vi "TwoPointCaculateAngle.vi"(2 "Point 2":cluster{"X":dbl, "Y":dbl}, 3 "Point 1":cluster{"X":dbl, "Y":dbl}) -> (0 "©·«×":dbl, 1 "deg( «×)":dbl)   [LabVIEW 2014]
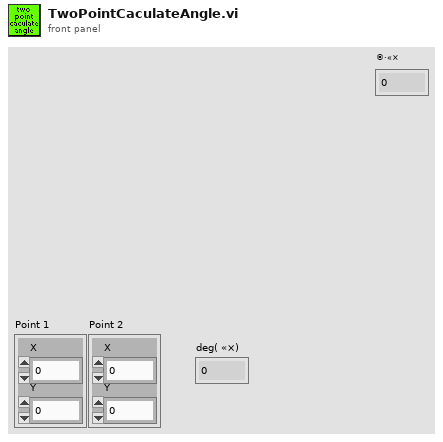
[diagram p1: front panel]
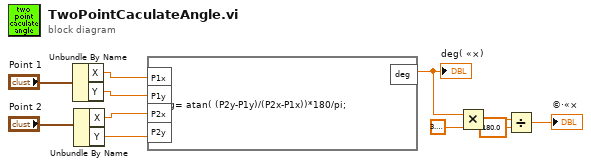
[diagram p0: block diagram]
diagram:
  n1 = Unbundle By Name("Point 1") -> ("X"=w9:dbl, "Y"=w8:dbl)
  n2 = Unbundle By Name("Point 2") -> ("X"=w7:dbl, "Y"=w6:dbl)
  n3 = formula code="deg= atan( (P2y-P1y)/(P2x-P1x))*180/pi;"("P1x"=w9, "P1y"=w8, "P2x"=w7, "P2y"=w6) -> ("deg"=w5:dbl)
  "deg( «×)" <- w5
  n4 = Multiply(x=w5, y=3.141592653589793) -> (x*y=w3:dbl)
  n5 = Divide(x=w3, y=180.0) -> (x/y=→"©·«×":dbl)
